vi "Add State(s) to Queue By BOOL(Array Left).vi"(4 "FALSE (\"\")":string, 6 "TRUE (\"\")":string[](array[string]), 8 "High Priority? (F)":bool, 10 "Condition":bool, 11 "State Queue (\"\")":string) -> (3 "Remaining States":string)   [LabVIEW 2017, in "Communicable State Machine.lvlib"]
doc: "Merges CSM message strings into the CSM message queue. This VI provides string options for both TRUE and FALSE states, avoiding the use of case structures and improving code readability and programming efficiency.\n\n\n> [!NOTE] <b>CSM State Queue Operation API</b>\n>\n> This type of API only concatenates message strings and does not send messages directly. The message is sent and the operation executed within the Parse State Queue++ VI. Unlike the Message Building API, this type of API includes a CSM state queue string input, which is equivalent to inserting a message into the state queue.\n\n\n-- <b>Controls</b> --\n- <b>State Queue (\"\")</b>: The entire state queue is connected to this input.\n- <b>Condition</b>: Selects the state string connected to the TRUE or FALSE terminal.\n- <b>High Priority? (F)</b>: If TRUE, the state is inserted at the front of the <b>State Queue (\"\")</b>. If FALSE, the state is appended to the end.\n- <b>TRUE (\"\")</b>: The state string to insert when <b>Condition</b> is TRUE.\n- <b>FALSE (\"\")</b>: The state string to insert when <b>Condition</b> is FALSE.\n\n-- <b>Indicators</b> --\n- <b>Remaining States</b>: Returns all concatenated states and arguments."
uses:
  Communicable State Machine.lvlib
  _Shared/CSM Shared.lvlib
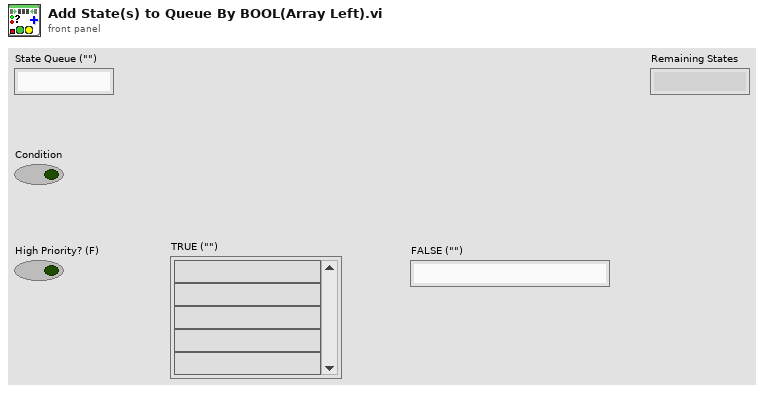
[diagram p1: front panel]
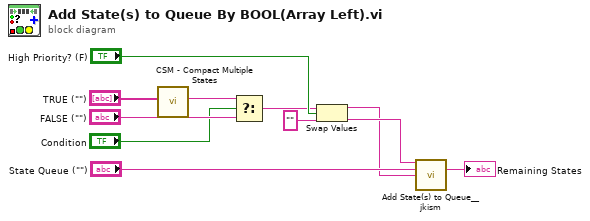
[diagram p0: block diagram]
diagram:
  n1 = call "CSM - Compact Multiple States.vi"("Multiple States"="TRUE (\"\")") -> ("States"=w1:string)  [unwired: 9 in]
  n2 = Select(t=w1, s="Condition", f="FALSE (\"\")") -> (s? t:f=w5:string)
  n3 = Swap Values(12:w5, 13:"High Priority? (F)", 14:"") -> (1:w2:string, 3:w3:string)
  n4 = call "Add State(s) to Queue__jkism.vi"("State(s) in Front (\"\")"=w3, "State(s) in (\"\")"="State Queue (\"\")", "State(s) at Back (\"\")"=w2) -> ("States Out"=→"Remaining States":string)  [unwired: 12 in]
